vi "lab3_abcd_nor.vi"() -> ()   [LabVIEW 2023]
panel:
  out ".not. (x .or. y)?":bool
  in  "d_in":bool
  in  "c_in":bool
  in  "b_in":bool
  in  "a_in":bool
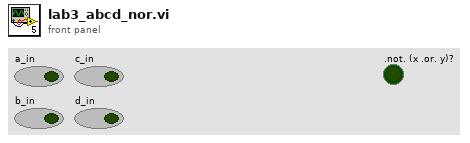
[diagram p1: front panel]
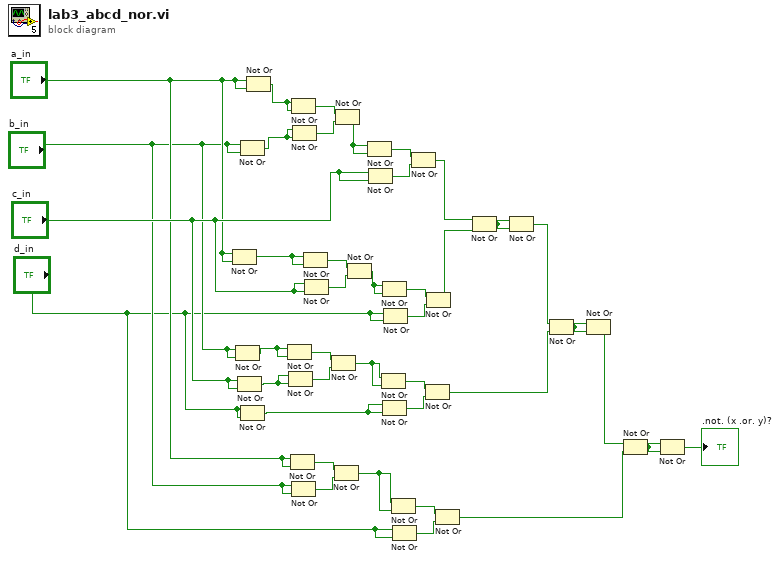
[diagram p0: block diagram]
diagram:
  n1 = Not Or(1:"a_in", 2:"a_in") -> (0:w31:bool)
  n2 = Not Or(1:"b_in", 2:"b_in") -> (0:w21:bool)
  n3 = Not Or(1:"c_in", 2:"c_in") -> (0:w20:bool)
  n4 = Not Or(1:"b_in", 2:"b_in") -> (0:w37:bool)
  n5 = Not Or(1:"d_in", 2:"d_in") -> (0:w16:bool)
  n6 = Not Or(1:"a_in", 2:"a_in") -> (0:w38:bool)
  n7 = Not Or(1:w21, 2:w21) -> (0:w23:bool)
  n8 = Not Or(1:w20, 2:w20) -> (0:w22:bool)
  n9 = Not Or(1:"a_in", 2:"a_in") -> (0:w15:bool)
  n10 = Not Or(1:w38, 2:w38) -> (0:w40:bool)
  n11 = Not Or(1:"b_in", 2:"b_in") -> (0:w14:bool)
  n12 = Not Or(1:w37, 2:w37) -> (0:w39:bool)
  n13 = Not Or(1:w31, 2:w31) -> (0:w33:bool)
  n14 = Not Or(1:"c_in", 2:"c_in") -> (0:w32:bool)
  n15 = Not Or(1:w22, 2:w23) -> (0:w17:bool)
  n16 = Not Or(1:w14, 2:w15) -> (0:w9:bool)
  n17 = Not Or(1:w39, 2:w40) -> (0:w34:bool)
  n18 = Not Or(1:w32, 2:w33) -> (0:w28:bool)
  n19 = Not Or(1:w34, 2:w34) -> (0:w36:bool)
  n20 = Not Or(1:"c_in", 2:"c_in") -> (0:w35:bool)
  n21 = Not Or(1:w17, 2:w17) -> (0:w19:bool)
  n22 = Not Or(1:w28, 2:w28) -> (0:w30:bool)
  n23 = Not Or(1:w16, 2:w16) -> (0:w18:bool)
  n24 = Not Or(1:"d_in", 2:"d_in") -> (0:w29:bool)
  n25 = Not Or(1:w9, 2:w9) -> (0:w11:bool)
  n26 = Not Or(1:"d_in", 2:"d_in") -> (0:w10:bool)
  n27 = Not Or(1:w35, 2:w36) -> (0:w26:bool)
  n28 = Not Or(1:w18, 2:w19) -> (0:w5:bool)
  n29 = Not Or(1:w29, 2:w30) -> (0:w27:bool)
  n30 = Not Or(1:w10, 2:w11) -> (0:w2:bool)
  n31 = Not Or(1:w27, 2:w26) -> (0:w25:bool)
  n32 = Not Or(1:w25, 2:w25) -> (0:w6:bool)
  n33 = Not Or(1:w5, 2:w6) -> (0:w7:bool)
  n34 = Not Or(1:w7, 2:w7) -> (0:w3:bool)
  n35 = Not Or(1:w2, 2:w3) -> (0:w4:bool)
  n36 = Not Or(1:w4, 2:w4) -> (0:→".not. (x .or. y)?":bool)
